vi "SaveAndCloseClassApp.vi"(8 "error in (no error)":errorcluster, 10 "Application":refnum<vi>, 11 "LVClassLibrary Ref":refnum<vi>) -> (0 "error out":errorcluster)   [LabVIEW 2019, in "BlueUtilityScripts.lvlib"]
uses:
  BlueUtilityScripts.lvlib
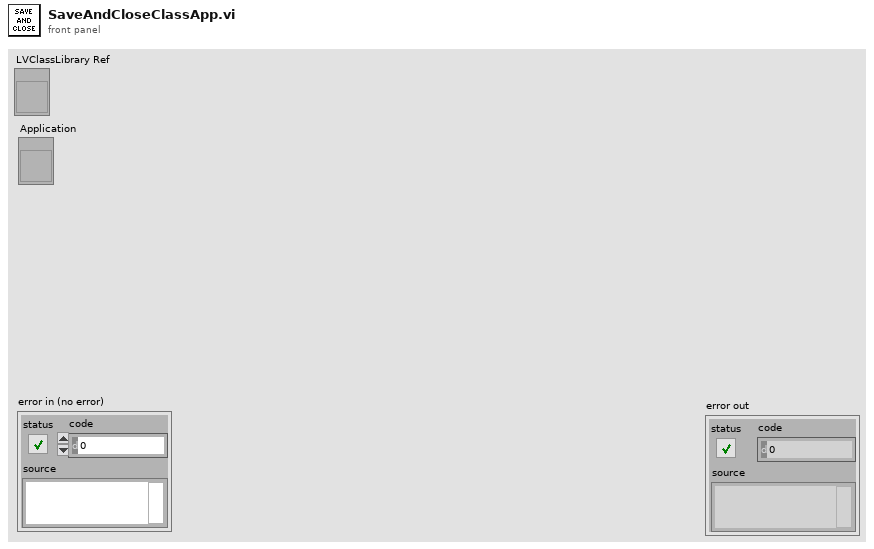
[diagram p1: front panel]
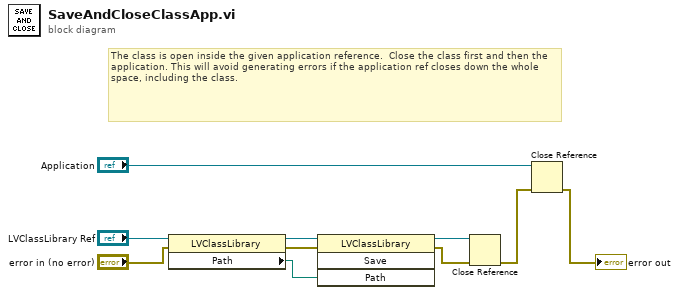
[diagram p0: block diagram]
diagram:
  # "The class is open inside the given application reference.  Close the class first and then the application. This will avoid generating errors if the application ref closes down the whole space, including the class."
  n1 = property class="LVClassLibrary"(reference="LVClassLibrary Ref", error in="error in (no error)") -> (reference out=w7:refnum<vi>, error out=w6:errorcluster, "Path"=w5:path)
  n2 = invoke class="LVClassLibrary" method="Save"(reference=w7, error in=w6, "Path"=w5) -> (reference out=w4:refnum<vi>, error out=w3:errorcluster)  [unwired: 1 in, 2 out]
  n3 = Close Reference(reference=w4, error in (no error)=w3) -> (error out=w2:errorcluster)
  n4 = Close Reference(reference="Application", error in (no error)=w2) -> (error out=→"error out":errorcluster)
